vi "ProdaNG.ProcessStepResult.Set.vi"(8 "error in (no error)":errorcluster, 9 "isRepeat (0)":i32, 10 "ProcessStepResult":T1, 11 "dbHandle":i32) -> (0 "error out":errorcluster, 3 "dbHandle":i32)   [LabVIEW 2016]
doc: "This function changes the process step result, which is defined by a ProcessStepResult structure. A process step result can either be set intentionally or leave the check of the test step results and the resulting changes to the DLL. In case, that the DLL changes the Process Result, the mdTime of the according Product is set to the current time and the mdProcessStepId is set to this process step. \nThe automatic check stands to the following rule:\n1. It is checked, if all test steps have the Status IO.\nIf the result of the test is IO, the status 1 (IO) is set in the test value result, otherwise the status 0 (NIO), respective 5 (IO Repeat) or 6 (NIO Repeat) in case of a repeat.\nParameter:\nhandle is an Integer, which is returned by the function Login() at the creation of a new connection.\nisRepeat shows, if this step is a repeat.\nprocessStepResult is a pointer on a ProcessStepResult structure, which elements must be prefilled. The structure must be defined and filled in the calling program. Changes can only be made on the elements StatusId, startTime and endTime. If the Endtime is not set, it is automatically filled with the current time by the DLL. \nThe element statusId is of particular importance:\nIf this element is passed with the value -1, the DLL makes a check on the test step results and sets the changeable elements automatically. Otherwise the returned values for status, start time and end time are set.\n\nReturncodes:\n0 No error\n< 0 ORACLE Error code\n6 (ERROR_INVALID_HANDLE) in case of an invalid handle\n1403 Record does not exist"
uses:
  Controls/ProdaNG.ProcessStepResult.ctl
  Controls/ProdaNG.ProcessStepResultSize.ctl
  prodllNG.dll
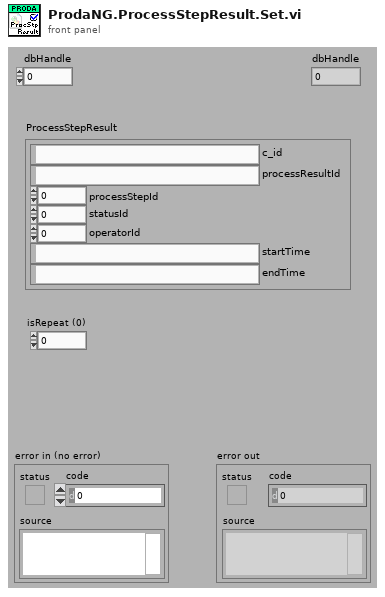
[diagram p1: front panel]
types:
  T1 = typedef "ProdaNG.ProcessStepResult.ctl" = cluster{"c_id":string, "processResultId":string, "processStepId":i32, "statusId":i32, "operatorId":i32, "startTime":string, "endTime":string}
  T2 = typedef "ProdaNG.ProcessStepResultSize.ctl" = cluster{"c_id":i32, "processResultId":i32, "processStepId":i32, "statusId":i32, "operatorId":i32, "startTime":i32, "endTime":i32}
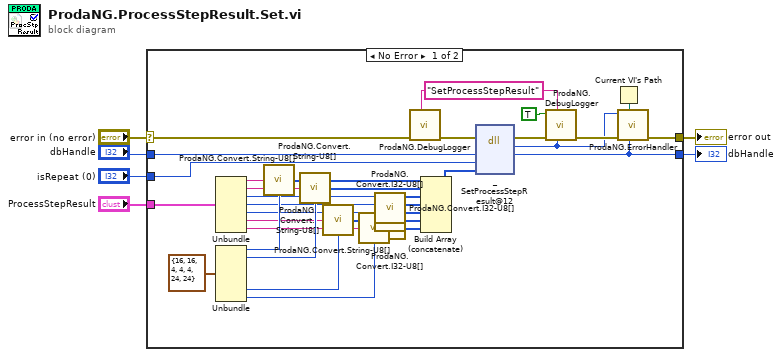
[diagram p0: block diagram]
diagram:
  n1 = case shown="No Error" "error in (no error)" {
    selector: "error in (no error)" -> [w21 w41]
    tunnel: [w8 w41] -> w5
    tunnel: [w7 w40] -> w4
    tunnel: "dbHandle" -> [w20 w40]
    tunnel: "isRepeat (0)" -> [w19 _]
    tunnel: "ProcessStepResult" -> [w18 _]
    frame No Error {
      w36 = "SetProcessStepResult" ("cmd")
      n2 = Unbundle(w18) -> ("c_id"=w38:string, "processResultId"=w39:string, "processStepId"=w26:i32, "statusId"=w25:i32, "operatorId"=w12:i32, "startTime"=w17:string, "endTime"=w16:string)
      n3 = Unbundle(T2 {"c_id"=16, "processResultId"=16, "processStepId"=4, "statusId"=4, "operatorId"=4, "startTime"=24, "endTime"=24} ("ProcessStepResultSize")) -> ("c_id"=w30:i32, "processResultId"=w28:i32, "startTime"=w10:i32, "endTime"=w9:i32)  [unwired: 3 out]
      n4 = call "ProdaNG.Convert.String-U8[].vi"("Input String"=w38, "Size"=w30) -> ("Output"=w29:u8[])
      n5 = call "ProdaNG.Convert.String-U8[].vi"("Input String"=w39, "Size"=w28) -> ("Output"=w27:u8[])
      n6 = call "ProdaNG.Convert.String-U8[].vi"("Input String"=w17, "Size"=w10) -> ("Output"=w14:u8[])
      n7 = call "ProdaNG.Convert.String-U8[].vi"("Input String"=w16, "Size"=w9) -> ("Output"=w15:u8[])
      n8 = call "ProdaNG.Convert.I32-U8[].vi"("32bit integer"=w26) -> ("unsigned byte array"=w24:u8[])  [unwired: 10 in]
      n9 = call "ProdaNG.Convert.I32-U8[].vi"("32bit integer"=w25) -> ("unsigned byte array"=w23:u8[])  [unwired: 10 in]
      n10 = call "ProdaNG.Convert.I32-U8[].vi"("32bit integer"=w12) -> ("unsigned byte array"=w13:u8[])  [unwired: 10 in]
      n11 = call "ProdaNG.DebugLogger.vi"("cmd"=w36, "error in (no error)"=w21) -> ("error out"=w31:errorcluster)  [unwired: 9 in]
      n12 = Build Array (concatenate)(w29, w27, w24, w23, w13, w14, w15) -> (w22:u8[])
      n13 = dll-call lib="D:/Maszup/WABCO/SVN/LineTraceSystem/SOFTWARE/sources/Database/ProdaNG/prodllNG.dll" fn="_SetProcessStepResult@12" ("ProDll.dll:InitProDll")(error in=w31, "dbHandle"=w20, "isRepeat"=w19, "processResult"=w22) -> (error out=w34:errorcluster, "return type"=w32:i32, "dbHandle"=w7:i32)  [unwired: 4 in, 1 out]
      n14 = call "ProdaNG.DebugLogger.vi"("return type"=w32, "cmd"=w36, "error in (no error)"=w34, "done? (F)"=TRUE) -> ("error out"=w33:errorcluster)  [unwired: 7 in]
      n15 = Current VI's Path() -> (path=w37:path)
      n16 = call "ProdaNG.ErrorHandler.vi"("dbHandleIn"=w7, "Path"=w37, "error in"=w33, "output_parameter"=w32) -> ("error out"=w8:errorcluster)  [unwired: 7 in]
    }
    frame Error {
    }
  }
  "error out" <- w5
  "dbHandle" <- w4
